vi "send_HVCriticalValues.vi"(4 "Counter":i32, 5 "200/freq":i32=10, 6 "Active":bool, 7 "CAN ID":u32=787 format="%x", 8 "Message":T2={"V_min [mV]"=3968.3673469387754, "T_max [C°]"=31.836734693877553, "Heartbeat"=0} {"T_max [C°]" scale=0.0..80.0; "V_min [mV]" scale=3000.0..4300.0}, 11 "CAN frame":T1[](array[typedef]) {"Data" format="%.0x"; "ArbitrationId" format="%.0x"; "Timestamp" format="%<%I:%M:%S%3u %p\n%m/%d/%Y>T"}) -> (3 "CAN frame out":T1[](array[typedef]) {"Data" format="%.0x"; "ArbitrationId" format="%.0x"; "Timestamp" format="%<%I:%M:%S%3u %p\n%m/%d/%Y>T"})   [LabVIEW 2017]
uses:
  <vilib>/nican/nican.llb/CanFrameTimed.ctl
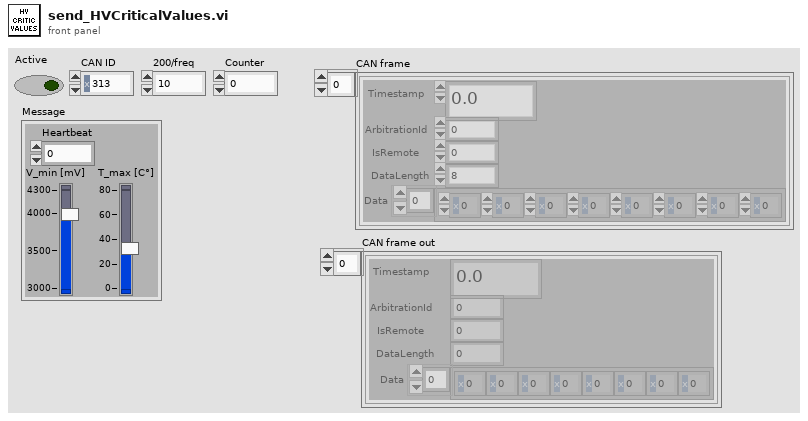
[diagram p1: front panel]
types:
  T1 = typedef "CanFrameTimed.ctl" = cluster{"Timestamp":dbl, "ArbitrationId":u32, "IsRemote":u8, "DataLength":u8, "Data":u8[]}
  T2 = cluster{"V_min [mV]":dbl, "T_max [C°]":dbl, "Heartbeat":u8}
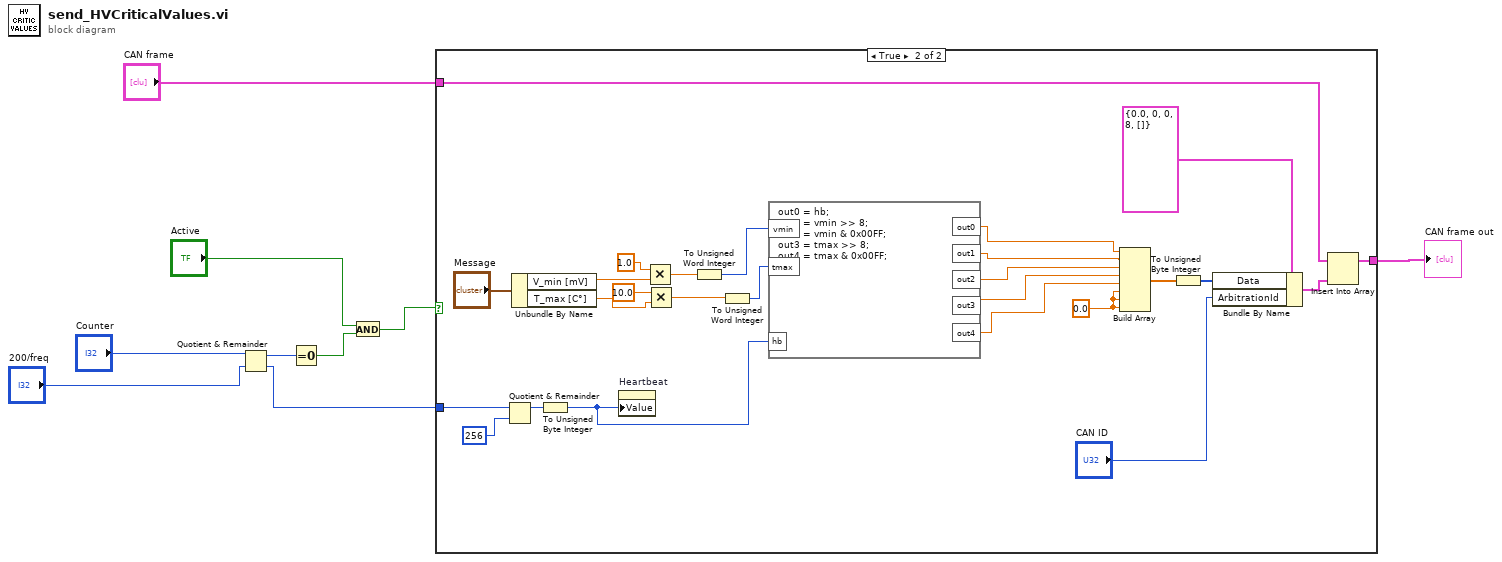
[diagram p0: block diagram]
diagram:
  n1 = Quotient & Remainder(x="Counter", y="200/freq") -> (x-y*floor(x/y)=w6:i32, floor(x/y)=w1:i32)
  n2 = Equal To 0?(x=w6) -> (x = 0?=w4:bool)
  n3 = And(x="Active", y=w4) -> (x .and. y?=w3:bool)
  n4 = case shown="True" w3 {
    tunnel: "CAN frame" -> [w10 w27]
    tunnel: [w10 w25] -> w8
    tunnel: w1 -> [_ w14]
    frame False {
    }
    frame True {
      w22 = 0.0 ("element")
      n5 = Quotient & Remainder(x=w14, y=256) -> (x-y*floor(x/y)=w12:i32)  [unwired: 1 out]
      n6 = Unbundle By Name("Message") -> ("V_min [mV]"=w21:dbl, "T_max [C°]"=w17:dbl)
      n7 = To Unsigned Byte Integer(number=w12) -> (unsigned 8bit integer=w11:u8)
      n8 = property on="Heartbeat" class="DigNum (strict)"("Value"=w11) -> ()  [unwired: 2 in, 2 out]
      n9 = Multiply(x=1.0, y=w21) -> (x*y=w20:dbl)
      n10 = Multiply(x=10.0, y=w17) -> (x*y=w16:dbl)
      n11 = To Unsigned Word Integer(number=w20) -> (unsigned 16bit integer=w23:u16)
      n12 = To Unsigned Word Integer(number=w16) -> (unsigned 16bit integer=w36:u16)
      n13 = formula code="out0 = hb;\nout1 = vmin >> 8;\nout2 = vmin & 0x00FF;\nout3 = tmax >> 8;\nout4 = tmax & 0x00FF;"("tmax"=w36, "hb"=w11, "vmin"=w23) -> ("out1"=w34:dbl, "out2"=w33:dbl, "out3"=w32:dbl, "out0"=w35:dbl, "out4"=w31:dbl)
      n14 = Build Array(w35, w34, w33, w32, w31, w22, w22, w22) -> (w30:dbl[])
      n15 = To Unsigned Byte Integer(number=w30) -> (unsigned 8bit integer=w29:u8[])
      n16 = Bundle By Name(cluster=T1 {"Timestamp"=0.0, "ArbitrationId"=0, "IsRemote"=0, "DataLength"=8, "Data"=[]} ("CAN frame"), "Data"=w29, "ArbitrationId"="CAN ID") -> (w26:T1)
      n17 = Insert Into Array(array=w27, new element=w26) -> (w25:T1[])  [unwired: 1 in]
    }
  }
  "CAN frame out" <- w8
